vi "SuppressBadChars.vi"(8 "error in (no error)":errorcluster, 11 "StringIn":string) -> (0 "error out":errorcluster, 3 "StringOut":string)   [LabVIEW 2011]
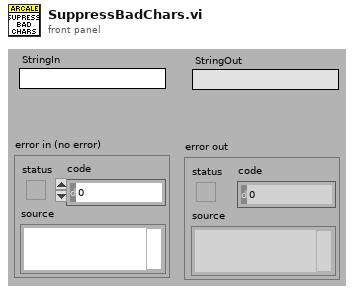
[diagram p1: front panel]
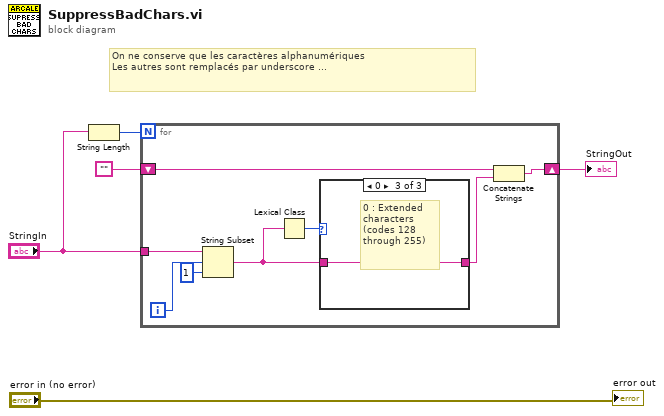
[diagram p0: block diagram]
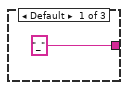
[diagram p2: hidden frame]
diagram:
  # "On ne conserve que les caractères alphanumériques\nLes autres sont remplacés par underscore ..."
  n1 = String Length(string="StringIn") -> (length=w5:i32)
  n2 = for {
    N: w5 -> [_]
    tunnel: "StringIn" -> [w13]
    shift-right: [w8] -> w2
    shift-left: "" -> [w6]
    i -> [w12]
    n3 = String Subset(string=w13, offset (0)=w12, length (rest)=1 ("length (rest)")) -> (substring=w9:string)
    n4 = Lexical Class(1:w9) -> (0:w10:i16)
    n5 = case shown="0" w10 {
      tunnel: w9 -> [_ w15 w16]
      tunnel: ["_" ("StringIn") w15 w16] -> w7
      frame Default {
      }
      frame 3..5 {
        # "3 : 0..9\n4 : A..Z\n5 : a..z"
      }
      frame 0 {
        # "0 : Extended \ncharacters \n(codes 128 \nthrough 255)"
      }
    }
    n6 = Concatenate Strings(w6, w7) -> (w8:string)
  }
  "StringOut" <- w2
  "error out" <- "error in (no error)"
